vi "Grab.vi"(6 "Reset":bool, 8 "Button Pressed?":bool, 9 "Arm Back?":bool, 10 "Arm Forward?":bool, 11 "Ball Present?":bool) -> (0 "Finished?":bool=TRUE, 2 "Arm state":T1, 3 "Roller Speed":dbl)   [LabVIEW 2013]
uses:
  <vilib>/Rock Robotics/WPI/Solenoid/WPI_SolenoidValue.ctl
  Grab States.ctl
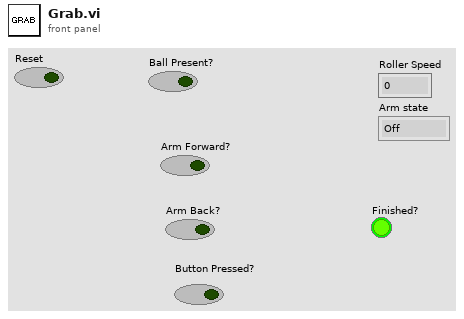
[diagram p1: front panel]
types:
  T1 = typedef "WPI_SolenoidValue.ctl" = enum16{"Off", "On", "Forward", "Reverse"}
  T2 = typedef "Grab States.ctl" = enum16{"Deploy Arm", "Wait for Ball", "Retract Arm"}
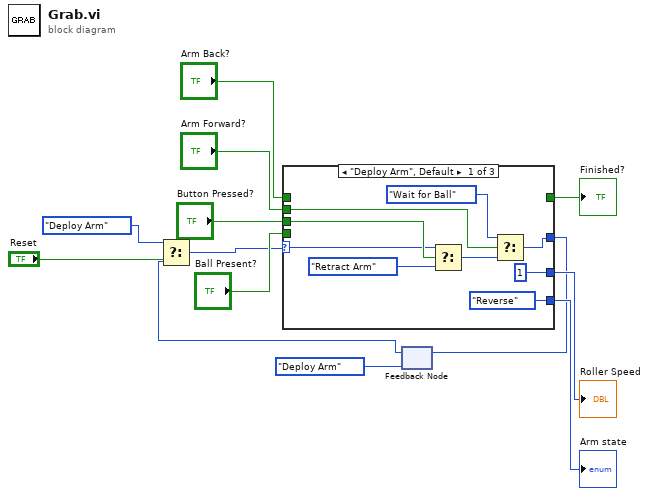
[diagram p0: block diagram]
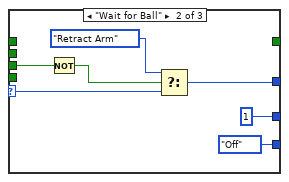
[diagram p2: hidden frame]
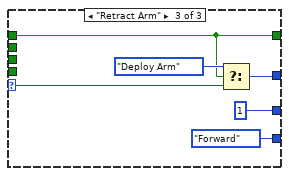
[diagram p3: hidden frame]
diagram:
  n1 = feedback #1(Grab_States."Deploy Arm" ("Grab VI State")) -> (w4:T2)
  n2 = Select(t=Grab_States."Deploy Arm" ("Grab VI State"), s="Reset", f=w4) -> (s? t:f=w5:T2)
  n3 = case shown="\"Deploy Arm\", Default" w5 {
    selector: w5 -> [w15 w26 w32]
    tunnel: [1 1 1] -> w12
    tunnel: [WPI_SolenoidValue."Reverse" ("Arm state") WPI_SolenoidValue."Off" ("Arm state") WPI_SolenoidValue."Forward" ("Arm state")] -> w11
    tunnel: "Arm Forward?" -> [w17 _ _]
    tunnel: [w18 w25 w31] -> w9
    tunnel: "Ball Present?" -> [_ _ _]
    tunnel: "Arm Back?" -> [_ _ w30]
    tunnel: "Button Pressed?" -> [w16 w24 _]
    tunnel: [_ _ w30] -> w1
    frame "Deploy Arm", Default {
      n4 = Select(t=w15, s=w16, f=Grab_States."Retract Arm" ("Grab VI State")) -> (s? t:f=w20:T2)
      n5 = Select(t=Grab_States."Wait for Ball" ("Grab VI State"), s=w17, f=w20) -> (s? t:f=w18:T2)
    }
    frame "Wait for Ball" {
      n6 = Not(x=w24) -> (.not. x?=w23:bool)
      n7 = Select(t=Grab_States."Retract Arm" ("Grab VI State"), s=w23, f=w26) -> (s? t:f=w25:T2)
    }
    frame "Retract Arm" {
      n8 = Select(t=Grab_States."Deploy Arm" ("Grab VI State"), s=w30, f=w32) -> (s? t:f=w31:T2)
    }
  }
  "Roller Speed" <- w12
  "Arm state" <- w11
  "Finished?" <- w1
  n9 = feedback-in #1(w9) -> ()
